vi "FYP_VI_MIDI_InstrumentData.vi"(1 "MIDI Channel":u32, 2 "Instrument":u32) -> (0 "MIDI Instrument data":u32)   [LabVIEW 2013]
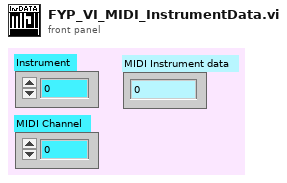
[diagram p1: front panel]
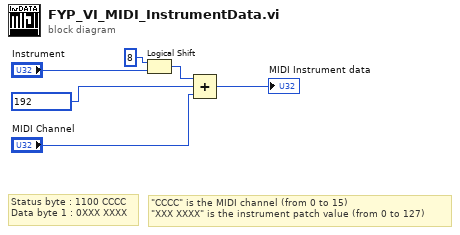
[diagram p0: block diagram]
diagram:
  # "\"CCCC\" is the MIDI channel (from 0 to 15)\n\"XXX XXXX\" is the instrument patch value (from 0 to 127)"
  # "Status byte : 1100 CCCC\nData byte 1 : 0XXX XXXX"
  n1 = Logical Shift(y=i16 8, x="Instrument") -> (x << y=w4:u32)
  n2 = Compound Arithmetic op=ADD(w4, u32 192 ("value"), "MIDI Channel") -> (→"MIDI Instrument data":u32)
